vi "ExShutterIN.vi"() -> ()   [LabVIEW 2010]
panel:
  out "Connection Open":bool
  in  "?":bool
  out "Shutter Is":string
  in  "?":bool
  in  "?":bool
  in  "?":bool
  out "error out":errorcluster
  in  "error in":errorcluster
  # "ExShutterIN.vi (InSpectrum Only)\nThis example shows how access the shutter on the InSpectrum.\nNOTE: The properly configured file SISpectActon.ini must be\npresent in the LabVIEW folder for spectrometer operation."
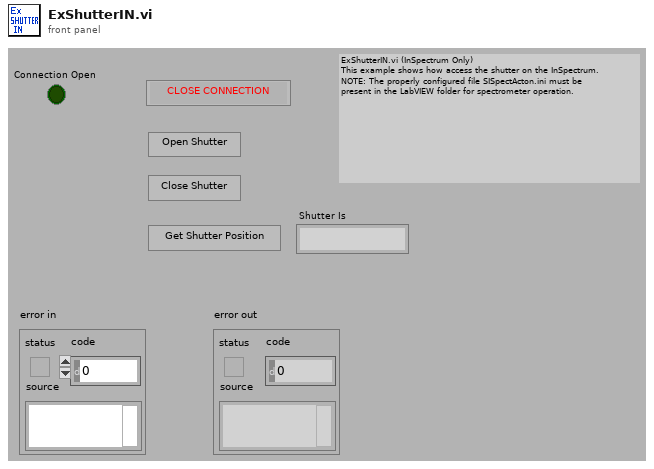
[diagram p1: front panel]
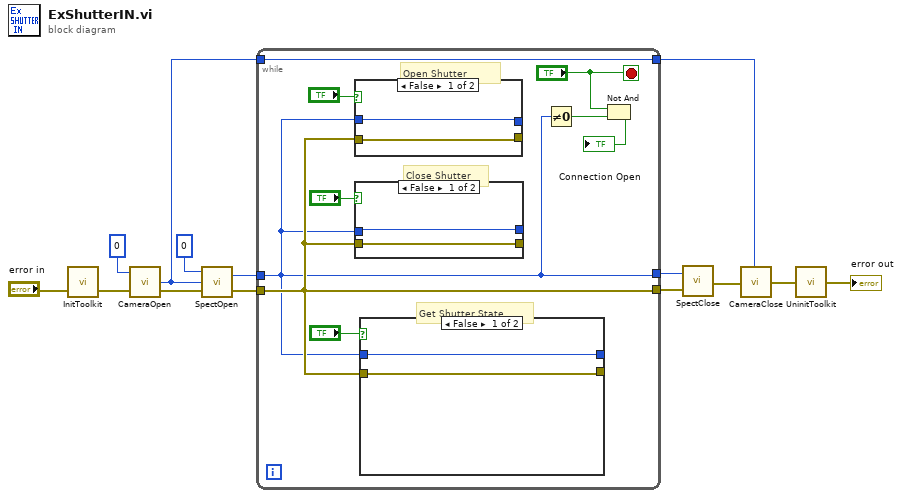
[diagram p0: block diagram]
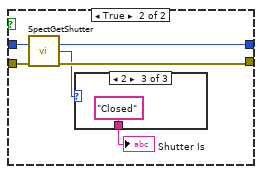
[diagram p2: hidden frame]
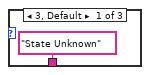
[diagram p3: hidden frame]
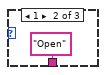
[diagram p4: hidden frame]
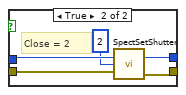
[diagram p5: hidden frame]
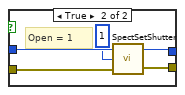
[diagram p6: hidden frame]
diagram:
  n1 = call <userlib>:"InitToolkit.vi"("error in"="error in") -> ("error out"=w6:errorcluster)
  n2 = call <userlib>:"CameraOpen.vi"("error in"=w6, "Camera Device ID"=0) -> ("error out"=w5:errorcluster, "Camera Handle"=w1:u32)
  n3 = call <userlib>:"SpectOpen.vi"("error in"=w5, "Camera Handle"=w1, "Spectrometer ID"=0) -> ("error out"=w11:errorcluster, "Spectrometer Handle"=w8:u32)
  n4 = while {
    tunnel: w8 -> [w15]
    tunnel: w11 -> [w16]
    tunnel: [w15] -> w10
    tunnel: [w16] -> w9
    tunnel: w1 -> [w17]
    tunnel: [w17] -> w2
    stop <- "?" stop-if-true
    # "Close Shutter"
    # "Open Shutter"
    # "Get Shutter State"
    n5 = case shown="False" "?" {
      tunnel: [w42 w48] -> _
      tunnel: [w43 w47] -> _
      tunnel: w15 -> [w43 w46]
      tunnel: w16 -> [w42 w45]
      frame False {
      }
      frame True {
        # "Open = 1"
        n6 = call <userlib>:"SpectSetShutter.vi"("error in"=w45, "State"=1, "Spectrometer Handle"=w46) -> ("error out"=w48:errorcluster, "Spectrometer Handle"=w47:u32)
      }
    }
    n7 = case shown="False" "?" {
      tunnel: w15 -> [w36 w41]
      tunnel: w16 -> [w35 w40]
      tunnel: [w35 w39] -> _
      tunnel: [w36 w38] -> _
      frame False {
      }
      frame True {
        # "Close = 2"
        n8 = call <userlib>:"SpectSetShutter.vi"("error in"=w40, "State"=2, "Spectrometer Handle"=w41) -> ("error out"=w39:errorcluster, "Spectrometer Handle"=w38:u32)
      }
    }
    n9 = case shown="False" "?" {
      tunnel: w16 -> [w24 w30]
      tunnel: w15 -> [w25 w31]
      tunnel: [w25 w28] -> _
      tunnel: [w24 w29] -> _
      frame False {
      }
      frame True {
        n10 = call <userlib>:"SpectGetShutter.vi"("error in"=w30, "Spectrometer Handle"=w31) -> ("error out"=w29:errorcluster, "Position"=w27:i16, "Spectrometer Handle"=w28:u32)  [unwired: 1 in]
        n11 = case shown="2" w27 {
          tunnel: ["State Unknown" "Open" "Closed"] -> w26
          frame 3, Default {
          }
          frame 1 {
          }
          frame 2 {
          }
        }
        "Shutter Is" <- w26
      }
    }
    n12 = Not Equal To 0?(x=w15) -> (x != 0?=w20:bool)
    n13 = Not And(1:w20, 2:"?") -> (0:→"Connection Open":bool)
  }
  n14 = call <userlib>:"SpectClose.vi"("error in"=w9, "Spectrometer Handle"=w10) -> ("error out"=w4:errorcluster)
  n15 = call <userlib>:"CameraClose.vi"("error in"=w4, "Camera Handle"=w2) -> ("error out"=w3:errorcluster)
  n16 = call <userlib>:"UninitToolkit.vi"("error in"=w3) -> ("error out"=→"error out":errorcluster)
